vi "Example_FG.vi"() -> ()   [LabVIEW 2017]
uses:
  FG Simulator.lvlib
panel:
  in  "VISA resource name":refnum<visa-resource-name>="TCPIP::localhost::9998::SOCKET"
  in  "stop":bool
  out "FG_Connected":bool
  in  "FG_Ampl":dbl(knob)=1.0 caption="Amplitude [V]" min=0.0 max=10.0 step=0.1 scale=0.0..10.0
  in  "FG_Offset":dbl(knob) caption="DC Offset [V]" min=-5.0 max=5.0 step=0.1 scale=-5.0..5.0
  in  "FG_Freq":dbl(knob)=1.0 caption="Frequency [Hz]" min=1.0 max=100.0 step=0.1 scale=1.0..100.0
  in  "FG_Fstart":dbl=0.1 caption="Start [Hz]"
  in  "FG_Fstop":dbl=10.0 caption="Stop [Hz]"
  in  "FG_Fstep":dbl=0.1 caption="Step [Hz]"
  in  "FG_Tstep":dbl=1.0 caption="Step [s]"
  in  "FG_Mode":bool caption="Mode"
  in  "FG_NoiseAmpl":dbl=0.09999999999999964 caption="Noise [V]" min=0.01 max=2.0 step=0.01
  in  "FG_DCycle":dbl=50.0 caption="DutyCycle [%]" min=20.0 max=80.0 step=1.0
  in  "FG_Noise":bool caption="Noise"
  in  "FG_Shape":u16(ring) caption="Shape" items=["SIN", "TRI", "SQU", "SAW"]
  # "Function Generator"
  # "Sweep\nMode"
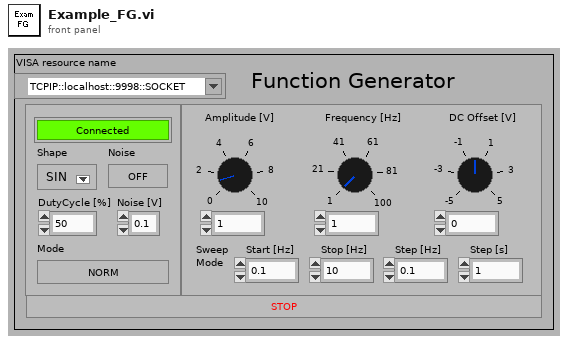
[diagram p1: front panel]
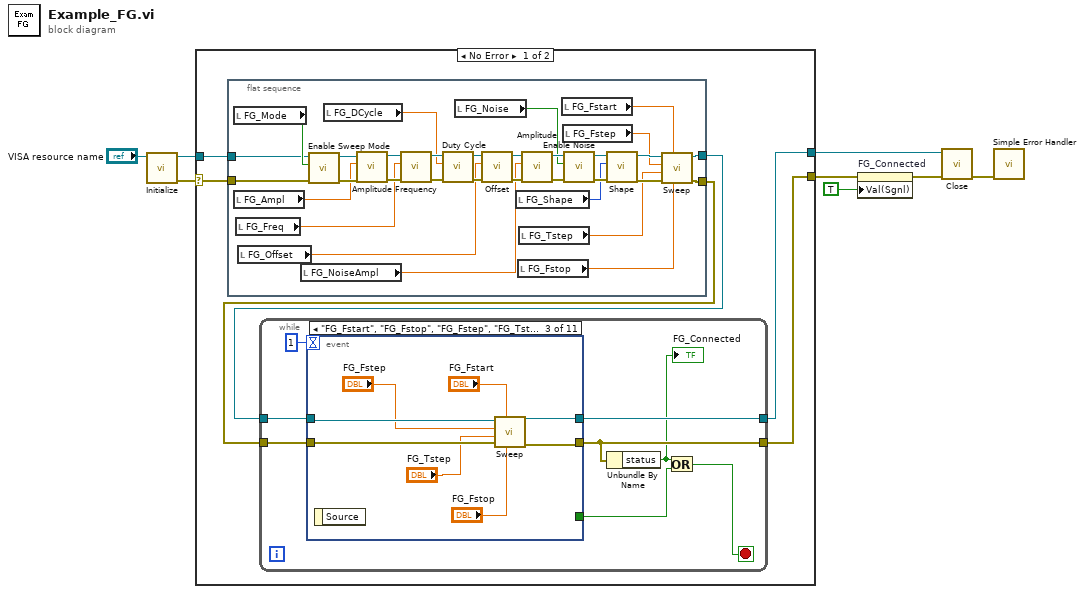
[diagram p0: block diagram]
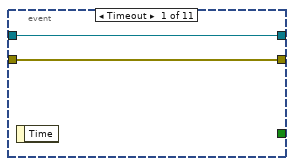
[diagram p2: hidden frame]
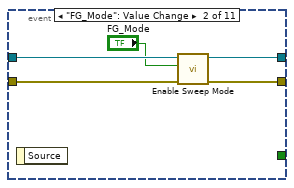
[diagram p3: hidden frame]
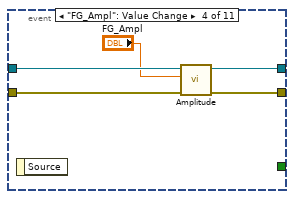
[diagram p4: hidden frame]
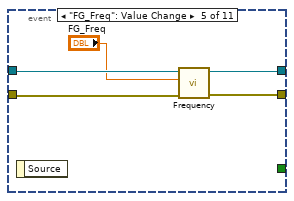
[diagram p5: hidden frame]
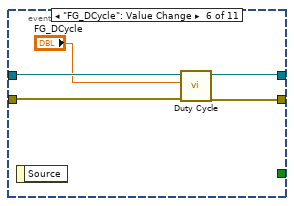
[diagram p6: hidden frame]
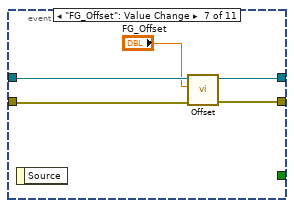
[diagram p7: hidden frame]
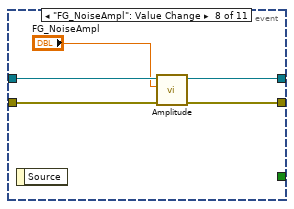
[diagram p8: hidden frame]
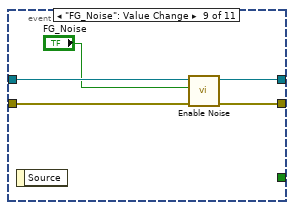
[diagram p9: hidden frame]
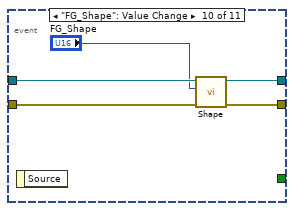
[diagram p10: hidden frame]
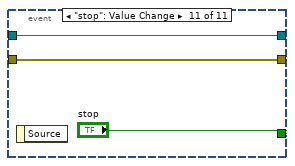
[diagram p11: hidden frame]
diagram:
  n1 = call "Initialize.vi"("VISA resource name"="VISA resource name") -> ("error out"=w6:errorcluster, "VISA resource name out"=w7:refnum<visa-resource-name>)  [unwired: 3 in, 6 out]
  n2 = case shown="No Error" w6 {
    selector: w6 -> [w9 w108]
    tunnel: [w14 w109] -> w8
    tunnel: [w13 w108] -> w5
    tunnel: w7 -> [w12 w109]
    frame No Error {
      n3 = flat-sequence {
        tunnel: w12 -> [w45]
        tunnel: w9 -> [w44]
        tunnel: [w27] -> w11
        tunnel: [w26] -> w10
        frame #0 {
          n4 = local read "FG_Mode"() -> (w46:bool)
          n5 = local read "FG_Ampl"() -> (w25:dbl)
          n6 = local read "FG_Freq"() -> (w24:dbl)
          n7 = local read "FG_Offset"() -> (w22:dbl)
          n8 = local read "FG_NoiseAmpl"() -> (w21:dbl)
          n9 = call "Enable Sweep Mode.vi"("error in (no error)"=w44, "Sweep (Off)"=w46, "VISA resource name"=w45) -> ("error out"=w43:errorcluster, "VISA resource name out"=w42:refnum<visa-resource-name>)  [unwired: 7 out]
          n10 = local read "FG_DCycle"() -> (w23:dbl)
          n11 = call "Amplitude.vi"("error in (no error)"=w43, "Amplitude (5)"=w25, "VISA resource name"=w42) -> ("error out"=w41:errorcluster, "VISA resource name out"=w40:refnum<visa-resource-name>)  [unwired: 7 out]
          n12 = call "Frequency.vi"("error in (no error)"=w41, "Frequency (5)"=w24, "VISA resource name"=w40) -> ("error out"=w39:errorcluster, "VISA resource name out"=w38:refnum<visa-resource-name>)  [unwired: 7 out]
          n13 = call "Duty Cycle.vi"("error in (no error)"=w39, "Duty Cycle (50)"=w23, "VISA resource name"=w38) -> ("error out"=w37:errorcluster, "VISA resource name out"=w36:refnum<visa-resource-name>)  [unwired: 7 out]
          n14 = local read "FG_Noise"() -> (w20:bool)
          n15 = call "Offset.vi"("error in (no error)"=w37, "Offset (5)"=w22, "VISA resource name"=w36) -> ("error out"=w35:errorcluster, "VISA resource name out"=w34:refnum<visa-resource-name>)  [unwired: 7 out]
          n16 = local read "FG_Shape"() -> (w19:u16)
          n17 = local read "FG_Fstop"() -> (w15:dbl)
          n18 = local read "FG_Tstep"() -> (w16:dbl)
          n19 = call "Amplitude.vi"("error in (no error)"=w35, "Amplitude (5)"=w21, "VISA resource name"=w34) -> ("error out"=w33:errorcluster, "VISA resource name out"=w32:refnum<visa-resource-name>)  [unwired: 7 out]
          n20 = local read "FG_Fstart"() -> (w18:dbl)
          n21 = local read "FG_Fstep"() -> (w17:dbl)
          n22 = call "Enable Noise.vi"("error in (no error)"=w33, "Noise (Off)"=w20, "VISA resource name"=w32) -> ("error out"=w31:errorcluster, "VISA resource name out"=w30:refnum<visa-resource-name>)  [unwired: 7 out]
          n23 = call "Shape.vi"("error in (no error)"=w31, "Shape"=w19, "VISA resource name"=w30) -> ("error out"=w28:errorcluster, "VISA resource name out"=w29:refnum<visa-resource-name>)  [unwired: 7 out]
          n24 = call "Sweep.vi"("Stop (10)"=w15, "Start (1)"=w18, "error in (no error)"=w28, "Dwell Time (1)"=w16, "Step (1)"=w17, "VISA resource name"=w29) -> ("error out"=w26:errorcluster, "VISA resource name out"=w27:refnum<visa-resource-name>)  [unwired: 4 in]
        }
      }
      n25 = while {
        tunnel: w11 -> [w53]
        tunnel: w10 -> [w54]
        tunnel: [w52] -> w14
        tunnel: [w51] -> w13
        stop <- w49 stop-if-true
        n26 = event shown="[2] \"FG_Fstart\", \"FG_Fstop\", \"FG_Fstep\", \"FG_Tstep\": Value Change" {
          selector: _ -> [_ _ _ _ _ _ _ _ _ _ _]
          dyn-events: _ -> [_ _ _ _ _ _ _ _ _ _ _]
          timeout: 1 -> [_ _ _ _ _ _ _ _ _ _ _]
          tunnel: w54 -> [w55 w58 w68 w71 w76 w81 w86 w91 w96 w101 w107]
          tunnel: w53 -> [w56 w59 w69 w74 w79 w84 w89 w94 w99 w104 w106]
          tunnel: [w56 w60 w66 w73 w78 w83 w88 w93 w98 w103 w106] -> w52
          tunnel: [w55 w61 w67 w72 w77 w82 w87 w92 w97 w102 w107] -> w51
          tunnel: [_ _ _ _ _ _ _ _ _ _ "stop"] -> w50
          event Timeout {
            n27 = event-data() -> ()  [unwired: 2 out]
          }
          event "FG_Mode": Value Change {
            n28 = event-data() -> ()  [unwired: 2 out]
            n29 = call "Enable Sweep Mode.vi"("error in (no error)"=w58, "Sweep (Off)"="FG_Mode", "VISA resource name"=w59) -> ("error out"=w61:errorcluster, "VISA resource name out"=w60:refnum<visa-resource-name>)  [unwired: 7 out]
          }
          event "FG_Fstart", "FG_Fstop", "FG_Fstep", "FG_Tstep": Value Change {
            n30 = event-data() -> ()  [unwired: 2 out]
            n31 = call "Sweep.vi"("Stop (10)"="FG_Fstop", "Start (1)"="FG_Fstart", "error in (no error)"=w68, "Dwell Time (1)"="FG_Tstep", "Step (1)"="FG_Fstep", "VISA resource name"=w69) -> ("error out"=w67:errorcluster, "VISA resource name out"=w66:refnum<visa-resource-name>)  [unwired: 4 in]
          }
          event "FG_Ampl": Value Change {
            n32 = event-data() -> ()  [unwired: 2 out]
            n33 = call "Amplitude.vi"("error in (no error)"=w71, "Amplitude (5)"="FG_Ampl", "VISA resource name"=w74) -> ("error out"=w72:errorcluster, "VISA resource name out"=w73:refnum<visa-resource-name>)  [unwired: 7 out]
          }
          event "FG_Freq": Value Change {
            n34 = event-data() -> ()  [unwired: 2 out]
            n35 = call "Frequency.vi"("error in (no error)"=w76, "Frequency (5)"="FG_Freq", "VISA resource name"=w79) -> ("error out"=w77:errorcluster, "VISA resource name out"=w78:refnum<visa-resource-name>)  [unwired: 7 out]
          }
          event "FG_DCycle": Value Change {
            n36 = event-data() -> ()  [unwired: 2 out]
            n37 = call "Duty Cycle.vi"("error in (no error)"=w81, "Duty Cycle (50)"="FG_DCycle", "VISA resource name"=w84) -> ("error out"=w82:errorcluster, "VISA resource name out"=w83:refnum<visa-resource-name>)  [unwired: 7 out]
          }
          event "FG_Offset": Value Change {
            n38 = event-data() -> ()  [unwired: 2 out]
            n39 = call "Offset.vi"("error in (no error)"=w86, "Offset (5)"="FG_Offset", "VISA resource name"=w89) -> ("error out"=w87:errorcluster, "VISA resource name out"=w88:refnum<visa-resource-name>)  [unwired: 7 out]
          }
          event "FG_NoiseAmpl": Value Change {
            n40 = event-data() -> ()  [unwired: 2 out]
            n41 = call "Amplitude.vi"("error in (no error)"=w91, "Amplitude (5)"="FG_NoiseAmpl", "VISA resource name"=w94) -> ("error out"=w92:errorcluster, "VISA resource name out"=w93:refnum<visa-resource-name>)  [unwired: 7 out]
          }
          event "FG_Noise": Value Change {
            n42 = event-data() -> ()  [unwired: 2 out]
            n43 = call "Enable Noise.vi"("error in (no error)"=w96, "Noise (Off)"="FG_Noise", "VISA resource name"=w99) -> ("error out"=w97:errorcluster, "VISA resource name out"=w98:refnum<visa-resource-name>)  [unwired: 7 out]
          }
          event "FG_Shape": Value Change {
            n44 = event-data() -> ()  [unwired: 2 out]
            n45 = call "Shape.vi"("error in (no error)"=w101, "Shape"="FG_Shape", "VISA resource name"=w104) -> ("error out"=w102:errorcluster, "VISA resource name out"=w103:refnum<visa-resource-name>)  [unwired: 7 out]
          }
          event "stop": Value Change {
            n46 = event-data() -> ()  [unwired: 2 out]
          }
        }
        n47 = Unbundle By Name(w51) -> ("status"=w48:bool)
        "FG_Connected" <- w48
        n48 = Or(x=w48, y=w50) -> (x .or. y?=w49:bool)
      }
    }
    frame Error {
    }
  }
  n49 = property on="FG_Connected" class="Bool (strict)"(error in=w5, "Val(Sgnl)"=TRUE ("Value (Signaling)")) -> (error out=w3:errorcluster)  [unwired: 1 in, 1 out]
  n50 = call "Close.vi"("error in (no error)"=w3, "VISA resource name"=w8) -> ("error out"=w4:errorcluster)  [unwired: 9 out]
  n51 = call <vilib>:"Simple Error Handler.vi"("error in (no error)"=w4) -> ()  [unwired: 1 in, 8 out]
